vi "G Type to PLC Type.vi"(9 "error in (no error)":errorcluster, 10 "Variant In":variant) -> (1 "error out":errorcluster, 3 "PLC Type":T1)   [LabVIEW 2018, in "TwinCAT ADS.lvclass"]
uses:
  TwinCAT ADS.lvclass
  Controls/PLC Type.ctl
  <vilib>/Utility/Data Type/NI_Data Type.lvlib
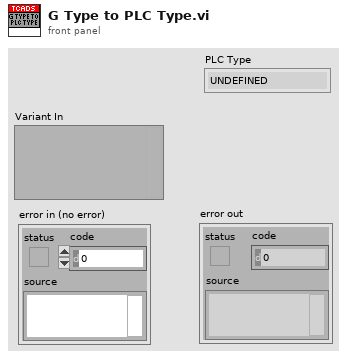
[diagram p1: front panel]
types:
  T1 = typedef "TwinCAT ADS.lvclass/PLC Type.ctl" = enum16{"UNDEFINED", "INT", "DINT", "REAL", "LREAL", "SINT", "BYTE", "UINT", "UDINT", "LINT", "ULINT", "STRING", "WSTRING", "BOOL", "TIME", "LTIME", "DATE", "DT", "TOD", "ARRAY", "JAGGED ARRAY", "STRUCT", "FUNCTION BLOCK", "UNION", "POINTER", "USER DEFINED"}
  T2 = typedef "NI_Data Type.lvlib/Data Type.ctl" = enum8{"Invalid Type", "Void", "I8", "I16", "I32", "I64", "U8", "U16", "U32", "U64", "Single Float", "Double Float", "Extended Float", "Single Complex", "Double Complex", "Extended Complex", "Enum U8", "Enum U16", "Enum U32", "Enum U64", "Single Float With Unit", "Double Float With Unit", "Extended Float With Unit", "Single Complex with Unit", "Double Complex with Unit", "Extended Complex with Unit", "Boolean", "String", "Path", "Picture", "Tag", "Array", "Cluster", "Variant", "LV Variant", "Waveform", "Timestamp", "Digital Waveform", "Digital Data", "ExpressData", "Refnum", "External Data", "VI", "Poly VI", "LabVIEW Class Instance", "Fixed Point"}
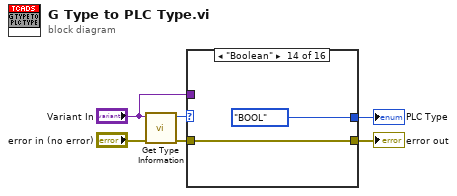
[diagram p0: block diagram]
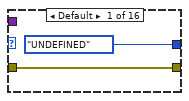
[diagram p2: hidden frame]
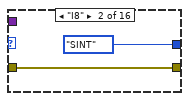
[diagram p3: hidden frame]
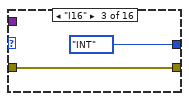
[diagram p4: hidden frame]
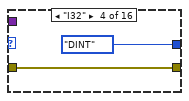
[diagram p5: hidden frame]
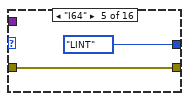
[diagram p6: hidden frame]
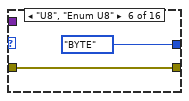
[diagram p7: hidden frame]
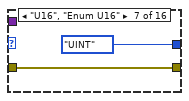
[diagram p8: hidden frame]
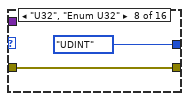
[diagram p9: hidden frame]
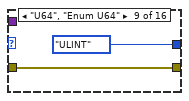
[diagram p10: hidden frame]
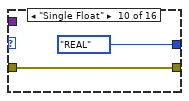
[diagram p11: hidden frame]
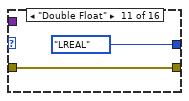
[diagram p12: hidden frame]
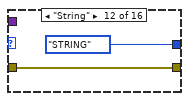
[diagram p13: hidden frame]
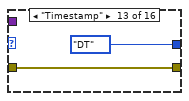
[diagram p14: hidden frame]
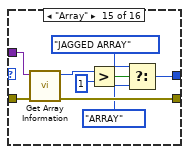
[diagram p15: hidden frame]
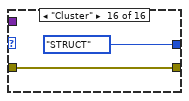
[diagram p16: hidden frame]
diagram:
  n1 = call <vilib>:"Get Type Information.vi"("error in (no error)"="error in (no error)", "Variant"="Variant In") -> ("error out"=w5:errorcluster, "Type"=w4:T2)  [unwired: 5 in, 3 out]
  n2 = case shown="\"Boolean\"" w4 {
    tunnel: w5 -> [w8 w10 w12 w14 w16 w18 w20 w22 w24 w26 w28 w30 w32 w34 w43 w45]
    tunnel: [w8 w10 w12 w14 w16 w18 w20 w22 w24 w26 w28 w30 w32 w34 w38 w45] -> w3
    tunnel: [PLC_Type."UNDEFINED" ("PLC Type") PLC_Type."SINT" ("PLC Type") PLC_Type."INT" ("PLC Type") PLC_Type."DINT" ("PLC Type") PLC_Type."LINT" ("PLC Type") PLC_Type."BYTE" ("PLC Type") PLC_Type."UINT" ("PLC Type") PLC_Type."UDINT" ("PLC Type") PLC_Type."ULINT" ("PLC Type") PLC_Type."REAL" ("PLC Type") PLC_Type."LREAL" ("PLC Type") PLC_Type."STRING" ("PLC Type") PLC_Type."DT" ("PLC Type") PLC_Type."BOOL" ("PLC Type") w35 PLC_Type."STRUCT" ("PLC Type")] -> w2
    tunnel: "Variant In" -> [_ _ _ _ _ _ _ _ _ _ _ _ _ _ w42 _]
    frame Default {
    }
    frame "I8" {
    }
    frame "I16" {
    }
    frame "I32" {
    }
    frame "I64" {
    }
    frame "U8", "Enum U8" {
    }
    frame "U16", "Enum U16" {
    }
    frame "U32", "Enum U32" {
    }
    frame "U64", "Enum U64" {
    }
    frame "Single Float" {
    }
    frame "Double Float" {
    }
    frame "String" {
    }
    frame "Timestamp" {
    }
    frame "Boolean" {
    }
    frame "Array" {
      n3 = call <vilib>:"Get Array Information.vi"("error in (no error)"=w43, "Variant"=w42) -> ("error out"=w38:errorcluster, "Number of Dimensions"=w41:i32)  [unwired: 6 in, 2 out]
      n4 = Greater?(x=w41, y=1) -> (0:w39:bool)
      n5 = Select(t=PLC_Type."JAGGED ARRAY" ("PLC Type"), s=w39, f=PLC_Type."ARRAY" ("PLC Type")) -> (s? t:f=w35:T1)
    }
    frame "Cluster" {
    }
  }
  "error out" <- w3
  "PLC Type" <- w2
